vi "DN4_CheckSamplesCountAndChannelsCount.vi"(1 "samples count":i32, 2 "channel count":i32) -> (0 "error out":errorcluster)   [LabVIEW 2020]
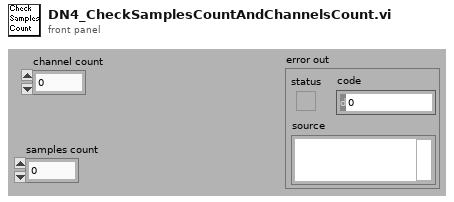
[diagram p1: front panel]
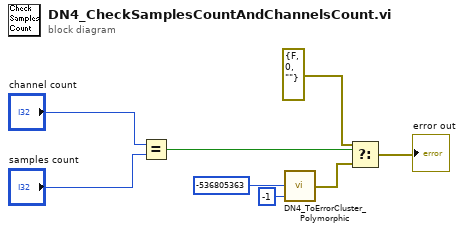
[diagram p0: block diagram]
diagram:
  n1 = Equal?(x="channel count", y="samples count") -> (x = y?=w6:bool)
  n2 = call "DN4_ToErrorCluster_Polymorphic.vi"("task id"=-1, "error code"=-536805363 ("error code (0)")) -> ("error out"=w2:errorcluster)  [unwired: 3 out]
  n3 = Select(t=errorcluster {"status"=FALSE, "code"=0, "source"=""}, s=w6, f=w2) -> (s? t:f=→"error out":errorcluster)
